vi "Log.vi"(8 "error in (no error)":errorcluster, 9 "Timestamp data points":bool, 10 "tdms file":refnum<k34>, 11 "Start Stream Result in":refnum<class "Start Stream Result.lvclass">) -> (0 "error out":errorcluster, 2 "tdms file out":refnum<k34>, 3 "Start Stream Result out":refnum<class "Start Stream Result.lvclass">)   [LabVIEW 2019, in "Start Stream Result.lvclass"]
uses:
  Start Stream Result.lvclass
  Acquired Result/Acquired Result.lvclass
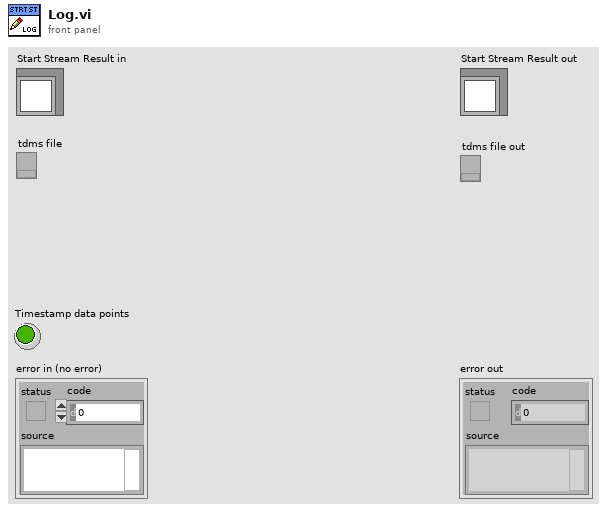
[diagram p1: front panel]
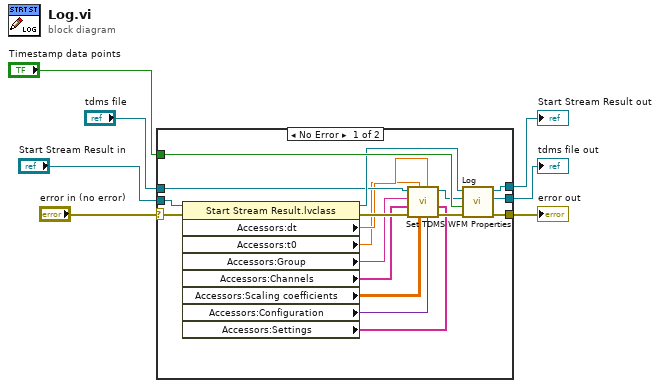
[diagram p0: block diagram]
diagram:
  n1 = case shown="No Error" "error in (no error)" {
    selector: "error in (no error)" -> [w10 w28]
    tunnel: [w25 w28] -> w7
    tunnel: [w24 w27] -> w6
    tunnel: [w23 w26] -> w5
    tunnel: "Timestamp data points" -> [w22 _]
    tunnel: "Start Stream Result in" -> [w19 w26]
    tunnel: "tdms file" -> [w16 w27]
    frame No Error {
      n2 = property class="Start Stream Result.lvclass"(reference=w19, error in=w10) -> (reference out=w18:refnum<class "Start Stream Result.lvclass">, error out=w20:errorcluster, "Accessors:dt"=w13:dbl, "Accessors:t0"=w12:dbl, "Accessors:Group"=w17:string, "Accessors:Channels"=w14:string[], "Accessors:Scaling coefficients"=w11:dbl[][], "Accessors:Configuration"=w9:variant, "Accessors:Settings"=w8:string[])
      n3 = call "Set TDMS WFM Properties.vi"("Settings"=w8, "Configuration"=w9, "dt"=w13, "Scaling coefficients"=w11, "t0"=w12, "error in (no error)"=w20, "Channel names"=w14, "Group name"=w17, "tdms file"=w16) -> ("error out"=w21:errorcluster, "tdms file out"=w15:refnum<k34>)  [unwired: 1 in]
      n4 = call-parent "Log.vi"("error in (no error)"=w21, "Timestamp data points"=w22, "tdms file"=w15, "Acquired Result in"=w18) -> ("error out"=w25:errorcluster, "tdms file out"=w24:refnum<k34>, "Acquired Result out"=w23:refnum<class "Start Stream Result.lvclass">)  [unwired: 5 in]
    }
    frame Error {
    }
  }
  "error out" <- w7
  "Start Stream Result out" <- w5
  "tdms file out" <- w6
